vi "Write Name.vi"(10 "Name":string, 11 "ITem":refnum<class "ITem.lvclass">) -> (3 "ITem In Out":refnum<class "ITem.lvclass">)   [LabVIEW 2020, in "ITem.lvclass"]
uses:
  ITem.lvclass
  ITem.lvclass/ITem.ctl
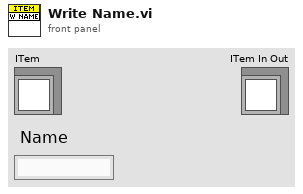
[diagram p1: front panel]
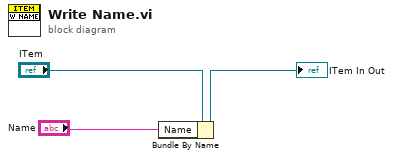
[diagram p0: block diagram]
diagram:
  n1 = Bundle By Name(cluster="ITem", "Name"="Name") -> (→"ITem In Out":refnum<class "ITem.lvclass">)
